vi "Autonomous_Thread.vi"   [LabVIEW 2015]
doc: "This VI is called when autonomous begins, and will automatically be terminated when autonomous ends. You can carry out timed or sensor driven robot movement independently without needing to return to the caller."
uses:
  <vilib>/Rock Robotics/Network Tables/NT Write String.vi
  Auto_Conf.vi
panel:
  # "Each item in this array is an autonomous script file.\nThis array is indexed by the autoMode variable in Robot Global Data."
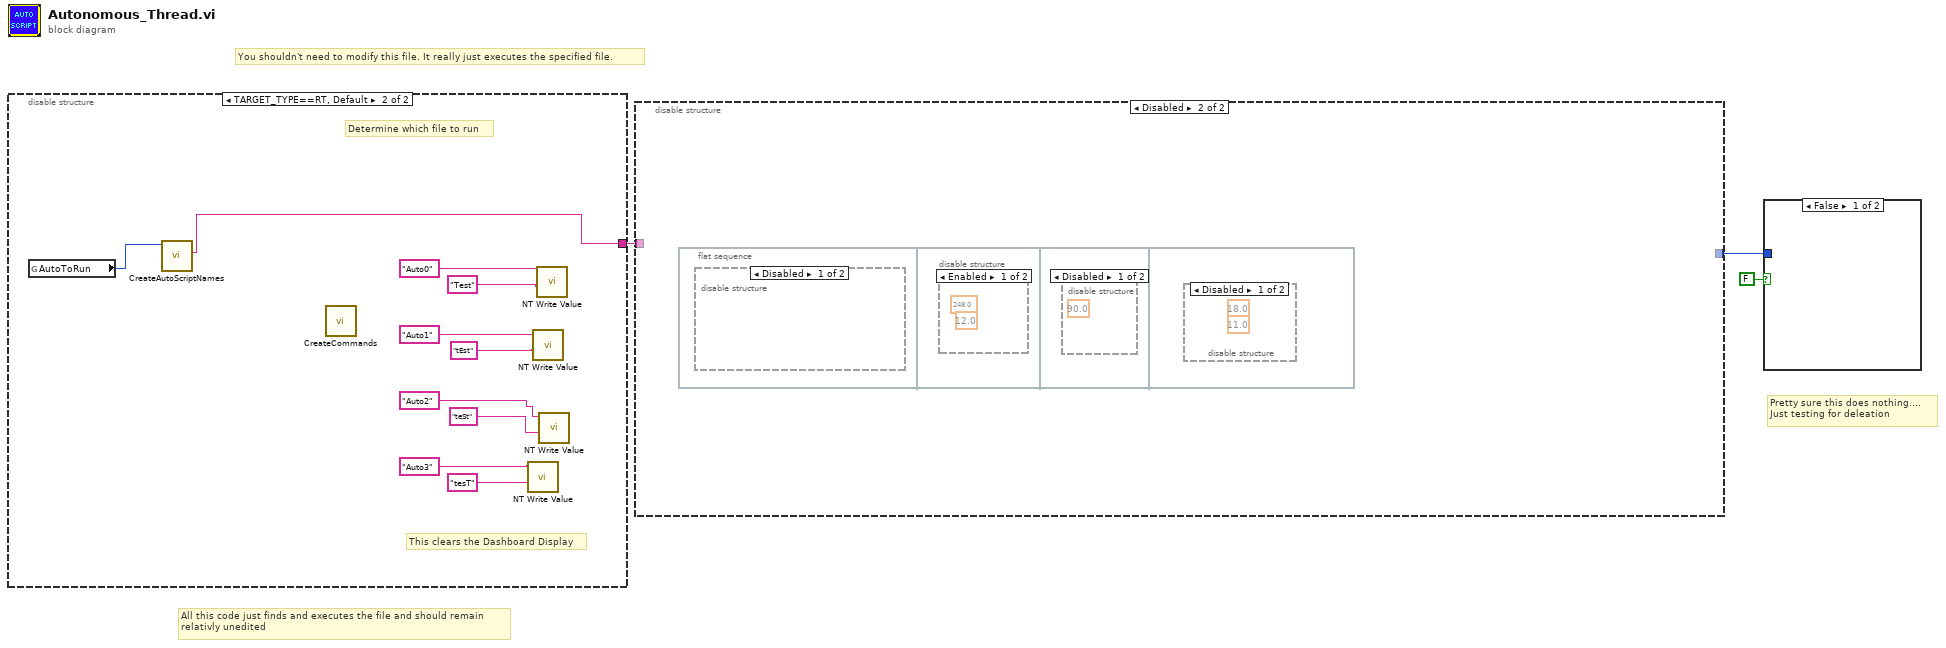
[diagram p0: block diagram]
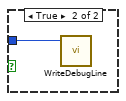
[diagram p2: hidden frame]
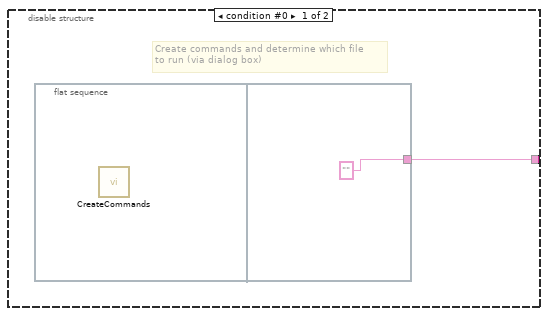
[diagram p3: hidden frame]
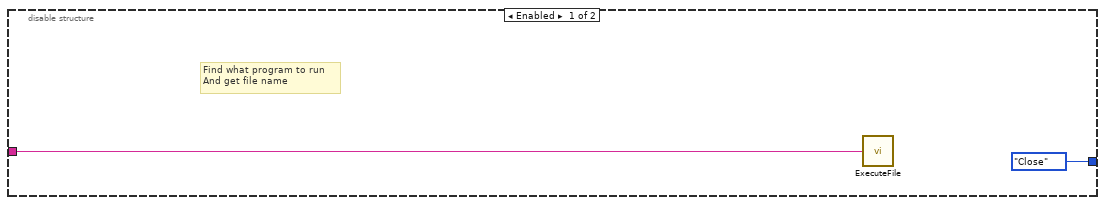
[diagram p4: hidden frame]
diagram:
  # "Pretty sure this does nothing.... \nJust testing for deleation"
  # "All this code just finds and executes the file and should remain\nrelativly unedited"
  # "You shouldn't need to modify this file. It really just executes the specified file."
  n1 = disable-structure shown="TARGET_TYPE==RT, Default" {
    disable-tunnel: [w4 w7] -> w3
    frame condition #0 {
      # "Create commands and determine which file\nto run (via dialog box)"
      n2 = flat-sequence {
        tunnel: ["" ("File Name With Extension")] -> w4
        frame #0 {
          n3 = call "CreateCommands.vi"() -> ()  [unwired: 1 out]
        }
        frame #1 {
        }
      }
    }
    frame condition #1 (active) {
      # "This clears the Dashboard Display"
      # "Determine which file to run"
      n4 = global read "Auto_Conf.vi" "AutoToRun"() -> (w6:u8)
      n5 = call "CreateAutoScriptNames.vi"("Index"=w6) -> ("Concat String"=w7:string)  [unwired: 10 in]
      n6 = call "CreateCommands.vi"() -> ()  [unwired: 1 in]
      n7 = call-poly <vilib>:"NT Write Value.vi"("String"="tesT", "Name"="Auto3") -> ()  [unwired: 9 in, 1 out]
      n8 = call-poly <vilib>:"NT Write Value.vi"("String"="tEst", "Name"="Auto1") -> ()  [unwired: 9 in, 1 out]
      n9 = call-poly <vilib>:"NT Write Value.vi"("String"="Test", "Name"="Auto0") -> ()  [unwired: 9 in, 1 out]
      n10 = call-poly <vilib>:"NT Write Value.vi"("String"="teSt", "Name"="Auto2") -> ()  [unwired: 9 in, 1 out]
    }
  }
  n11 = disable-structure shown="Disabled" {
    disable-tunnel: w3 -> [w17 _]
    disable-tunnel: [enum16{"Open", "Write Line", "Close"}."Close" ("Mode") _] -> w2
    frame Enabled {
      # "Find what program to run\nAnd get file name"
      n12 = call "ExecuteFile.vi"("File Name With Extension"=w17) -> ()
    }
    frame Disabled {
      n13 = flat-sequence {
        frame #0 {
          n14 = disable-structure shown="Disabled" {
            frame Disabled {
            }
            frame Enabled {
            }
          }
        }
        frame #1 {
          n15 = disable-structure shown="Enabled" {
            frame Enabled {
              (unwired) 248.0 ("Distance")
              (unwired) 12.0 ("Speed (ft/sec)")
            }
            frame Disabled {
            }
          }
        }
        frame #2 {
          n16 = disable-structure shown="Disabled" {
            frame Disabled {
              (unwired) 90.0 ("Angle")
            }
            frame Enabled {
            }
          }
        }
        frame #3 {
          n17 = disable-structure shown="Disabled" {
            frame Disabled {
              (unwired) 18.0 ("Distance")
              (unwired) 11.0 ("Speed (ft/sec)")
            }
            frame Enabled {
            }
          }
        }
      }
    }
  }
  n18 = case shown="False" FALSE {
    tunnel: w2 -> [_ w18]
    frame False {
    }
    frame True {
      n19 = call "WriteDebugLine.vi"("Mode"=w18) -> ()  [unwired: 1 in, 10 out]
    }
  }
